vi "UpdateVoffset.vi"(7 "LabVIEW Web Service Request":refnum<class "Web Request.lvclass">, 11 "Voffset":string) -> ()   [LabVIEW 2014]
uses:
  <vilib>/wsapi/Web Request.lvclass
  Controller/Controls/Enqueuer Enum.ctl
  Instr Actor/Messages/Set Voffset MSG/Set Voffset MSG.lvclass
  Instr Actor/Messages/Set Voffset MSG/Set Voffset MSG.lvclass/Set Voffset MSG.ctl
  Controller/Controller.lvclass
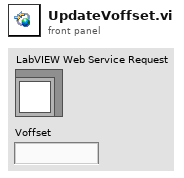
[diagram p1: front panel]
types:
  T1 = typedef "Controller.lvlib/Controller.lvclass/Enqueuer Enum.ctl" = enum8{"PAS", "CRDS", "File", "O3Lamp"}
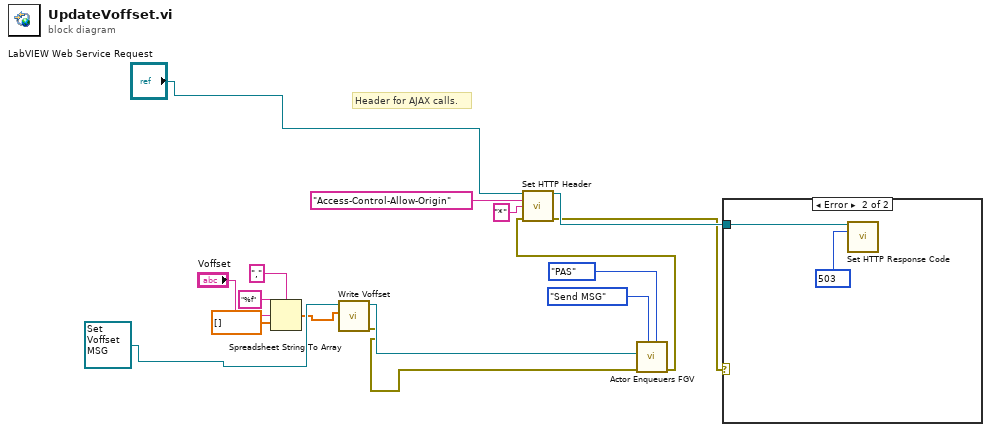
[diagram p0: block diagram]
diagram:
  # "Header for AJAX calls."
  n1 = Spreadsheet String To Array(delimiter (Tab)=",", format string="%f", spreadsheet string="Voffset", array type (2D Dbl)=dbl[] []) -> (array=w8:dbl[])
  n2 = call "Write Voffset.vi"("Voffset"=w8, "Set f0 MSG in"=refnum<class "Set Voffset MSG.lvclass"> refnum ("Instrument Lib:Set Voffset MSG.lvclass")) -> ("error out"=w7:errorcluster, "Set f0 MSG out"=w10:refnum<class "Set Voffset MSG.lvclass">)  [unwired: 8 in]
  n3 = call "Actor Enqueuers FGV.vi"("Enqueuer"=Enqueuer_Enum."PAS", "State"=enum16{"Store", "Send MSG"}."Send MSG", "error in"=w7, "MSG"=w10) -> ("error out"=w2:errorcluster)  [unwired: 7 in]
  n4 = call <vilib>:"Set HTTP Header.vi"("LabVIEW Web Service Request"="LabVIEW Web Service Request", "header"="Access-Control-Allow-Origin", "header value"="*", "error in (no error)"=w2) -> ("LabVIEW Web Service Request out"=w3:refnum<class "Web Request.lvclass">, "error out"=w1:errorcluster)  [unwired: 10 in]
  n5 = case shown="Error" w1 {
    tunnel: w3 -> [_ w17]
    frame No Error {
    }
    frame Error {
      w18 = 503 items=["100"=100, "101"=101, "200"=200, "201"=201, "202"=202, "203"=203, "204"=204, "205"=205, "206"=206, "300"=300, "301"=301, "302"=302, "303"=303, "304"=304, "305"=305, "306"=306, "307"=307, "400"=400, "401"=401, "402"=402, "403"=403, "404"=404, "405"=405, "406"=406, "407"=407, "408"=408, "409"=409, "410"=410, "411"=411, "412"=412, "413"=413, "414"=414, "415"=415, "416"=416, "417"=417, "500"=500, "501"=501, "502"=502, "503"=503, "504"=504, "505"=505] ("response code (200)")
      n6 = call <vilib>:"Set HTTP Response Code.vi"("LabVIEW Web Service Request"=w17, "response code (200)"=w18) -> ()  [unwired: 12 in, 2 out]
    }
  }
